vi "Get_Parameter Json.vi"(8 "error in (no error)":errorcluster caption="entrée d'erreur (pas d'erreur)", 11 "Class Instrument Firebase Altyor en entrée":refnum<class "Class Instrument Firebase Altyor.lvclass">) -> (0 "error out":errorcluster caption="sortie d'erreur", 2 "Parameter Json":string, 3 "Class Instrument Firebase Altyor en sortie":refnum<class "Class Instrument Firebase Altyor.lvclass">)   [LabVIEW 2020, in "Library Instrument & Equipement.lvlib" / "Library Instruments.lvlib" / "Class Instrument Firebase Altyor.lvclass"]
uses:
  Class Instrument Firebase Altyor.lvclass
  Class Instrument Firebase Altyor.lvclass/Class Instrument Firebase Altyor.ctl
  JSON API/Variant JSON/Variant to JSON.vi
  JSON API/JSON Value/Get Item by name array.vi
  Instrument (Default)/Class Instrument (Default).lvclass
  JSON API/JSON Value/JSON Value.lvclass
  JSON API/Get Polymorphic/JSON GetSet.lvlib
  JSON API/Variant JSON/Variant JSON.lvlib
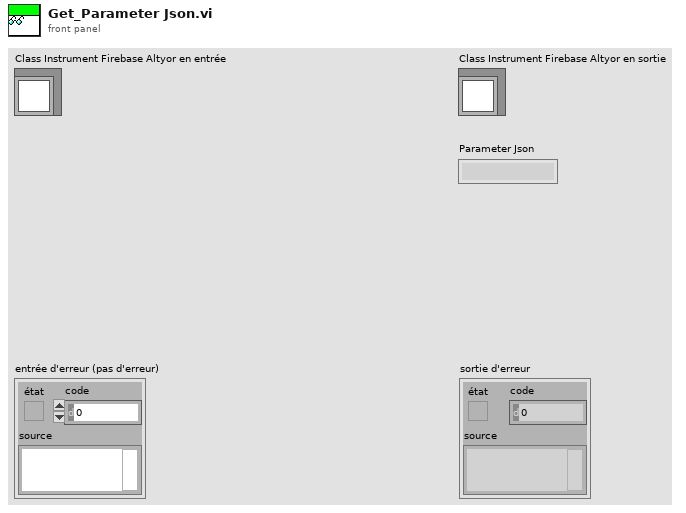
[diagram p1: front panel]
types:
  T1 = typedef "Library Commun.lvlib/Parameter Firebase Altyor.ctl" = cluster{"Name_BDD":string, "API_Key":string, "Nb_to_Read":string, "Value_to_find":string, "Field_Filter":string, "Field_Order":string, "Collection_to_find":string, "Name_Bench":string, "Bench Type":T2, "Type Data ":enum16{"Data Product", "Data Test"}, "Firebase Altyor":refnum<class "Firebase Altyor.lvclass">}
  T2 = typedef "Library Commun.lvlib/Bench Type.ctl" = enum16{"Bench PCBA", "Bench Camera", "Bench Assembly", "Bench PCBA P2193"}
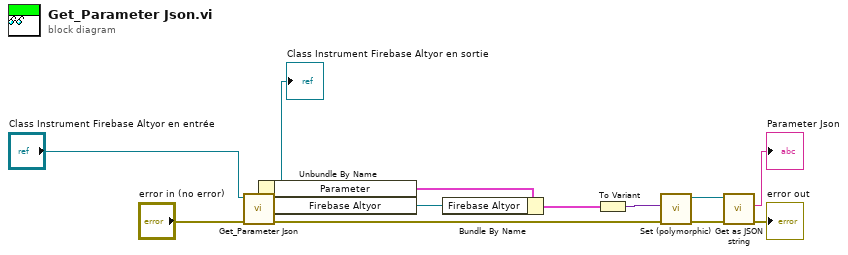
[diagram p0: block diagram]
diagram:
  n1 = call-parent "Get_Parameter Json.vi"("error in (no error)"="error in (no error)", "Class Instrument (Default) en entrée"="Class Instrument Firebase Altyor en entrée") -> ("error out"=w6:errorcluster, "Class Instrument (Default) en sortie"=w4:refnum<class "Class Instrument Firebase Altyor.lvclass">)  [unwired: 7 in, 1 out]
  "Class Instrument Firebase Altyor en sortie" <- w4
  n2 = Unbundle By Name(w4) -> ("Parameter"=w1:T1, "Firebase Altyor"=w3:refnum<class "Firebase Altyor.lvclass">)
  n3 = Bundle By Name(cluster=w1, "Firebase Altyor"=w3) -> (w2:T1)
  n4 = To Variant(anything=w2) -> (Variant=w10:variant)
  n5 = call-poly "Set (polymorphic).vi"("error in (no error)"=w6, "Variant"=w10) -> ("error out"=w8:errorcluster, "JSON Value out"=w9:refnum<class "JSON Value.lvclass">)  [unwired: 8 in]
  n6 = call "Get as JSON string.vi"("error in (no error)"=w8, "JSON Value in"=w9) -> ("error out"=→"error out":errorcluster, "<JSON>"=→"Parameter Json":string)  [unwired: 8 in]
